vi "All_Data_To_Cluster.vi"(0 "Test":sgl[][](array[numeric]), 1 "Dev":sgl[](array[numeric]), 2 "Inacc":sgl[](array[numeric]), 3 "DIN":string, 4 "HN":string[](array[string]), 5 "HS":sgl[](array[numeric]), 6 "TEMP":string, 7 "TV":sgl[][](array[numeric]), 8 "TSN":string, 9 "HV":sgl[](array[numeric]), 10 "MODE":string, 11 "REP":sgl[](array[numeric]), 13 "AVG":sgl[](array[numeric])) -> (14 "All_data_String":string[][](array[string]), 16 "Test_Data":T1)   [LabVIEW 2019]
uses:
  Test_data.ctl
  Test_load.ctl
  Hardness_test.ctl
  TEST.lvclass
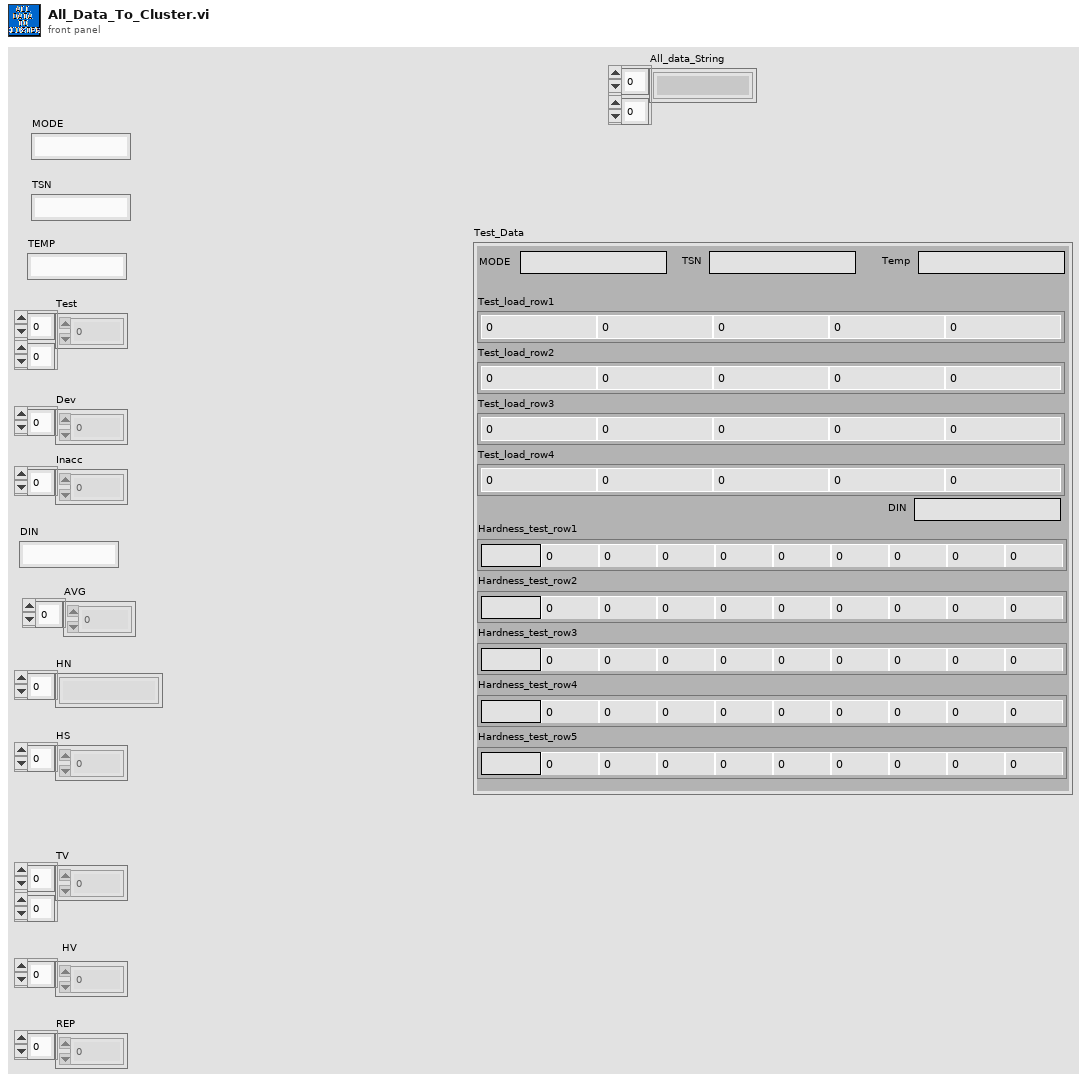
[diagram p1: front panel]
types:
  T1 = typedef "TEST.lvclass/Test_data.ctl" = cluster{"MODE":string, "TSN":string, "Temp":string, "Test_load_row1":T2, "Test_load_row2":T2, "Test_load_row3":T2, "Test_load_row4":T2, "DIN":string, "Hardness_test_row1":T3, "Hardness_test_row2":T3, "Hardness_test_row3":T3, "Hardness_test_row4":T3, "Hardness_test_row5":T3}
  T2 = typedef "TEST.lvclass/Test_load.ctl" = cluster{"TEST1":sgl, "TEST2":sgl, "TEST3":sgl, "DEV":sgl, "INACC":sgl}
  T3 = typedef "TEST.lvclass/Hardness_test.ctl" = cluster{"HN":string, "HS":sgl, "TV1":sgl, "TV2":sgl, "TV3":sgl, "TV4":sgl, "TV5":sgl, "AVG":sgl, "HV":sgl, "REP":sgl}
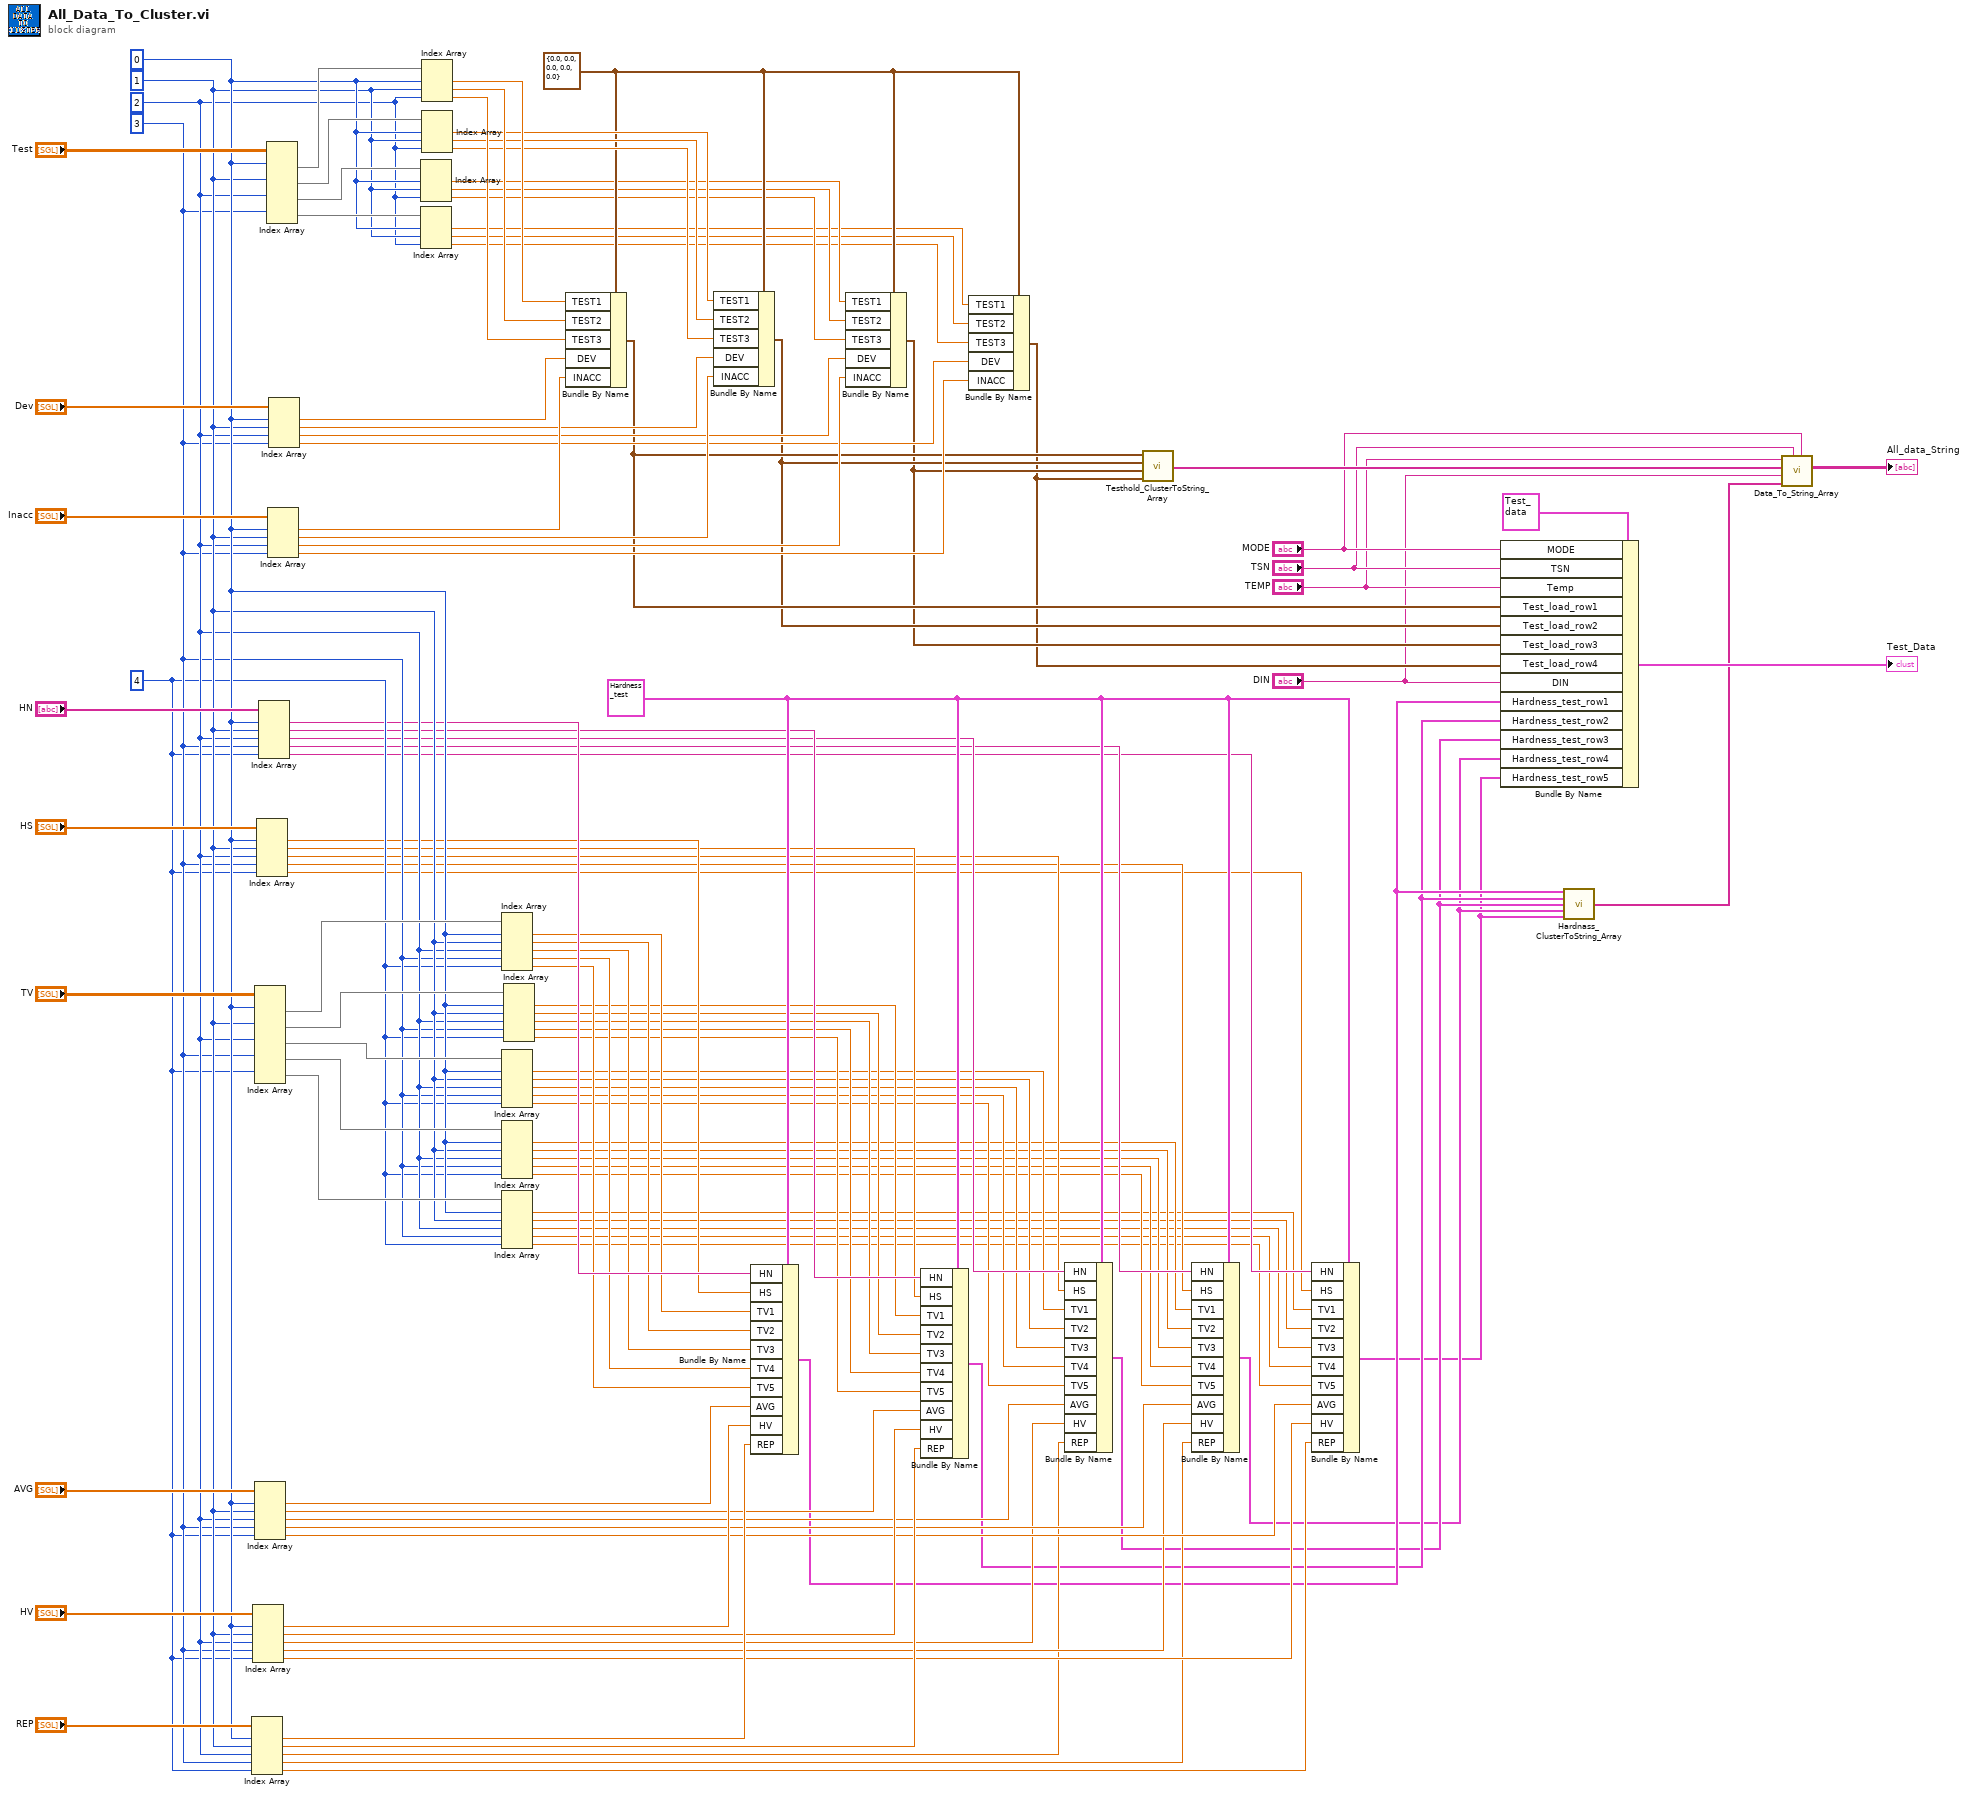
[diagram p0: block diagram]
diagram:
  w64 = T3 {"HN"="", "HS"=0.0, "TV1"=0.0, "TV2"=0.0, "TV3"=0.0, "TV4"=0.0, "TV5"=0.0, "AVG"=0.0, "HV"=0.0, "REP"=0.0} ("Hardness_test")
  w70 = 4
  w98 = T2 {"TEST1"=0.0, "TEST2"=0.0, "TEST3"=0.0, "DEV"=0.0, "INACC"=0.0} ("Test_load")
  w71 = 3 ("索引 (行)")
  w72 = 2 ("索引 (行)")
  w73 = 1 ("索引 (行)")
  w74 = 0 ("索引 (行)")
  n1 = Index Array(array="REP", index #1=w74, index #2=w73, index #3=w72, index #4=w71, index #5=w70) -> (element #1=w65:sgl, element #2=w59:sgl, element #3=w46:sgl, element #4=w45:sgl, element #5=w44:sgl)
  n2 = Index Array(array="HV", index #1=w74, index #2=w73, index #3=w72, index #4=w71, index #5=w70) -> (element #1=w66:sgl, element #2=w60:sgl, element #3=w49:sgl, element #4=w48:sgl, element #5=w47:sgl)
  n3 = Index Array(array="TV", index (row) #1=w74, index (row) #2=w73, index (row) #3=w72, index (row) #4=w71, index (row) #5=w70) -> (element #1=w79:sgl[], element #2=w78:sgl[], element #3=w77:sgl[], element #4=w76:sgl[], element #5=w75:sgl[])  [unwired: 5 in]
  n4 = Index Array(array="AVG", index #1=w74, index #2=w73, index #3=w72, index #4=w71, index #5=w70) -> (element #1=w67:sgl, element #2=w61:sgl, element #3=w52:sgl, element #4=w51:sgl, element #5=w50:sgl)
  n5 = Index Array(array="HS", index #1=w74, index #2=w73, index #3=w72, index #4=w71, index #5=w70) -> (element #1=w68:sgl, element #2=w62:sgl, element #3=w55:sgl, element #4=w54:sgl, element #5=w53:sgl)
  n6 = Index Array(array="HN", index #1=w74, index #2=w73, index #3=w72, index #4=w71, index #5=w70) -> (element #1=w69:string, element #2=w63:string, element #3=w58:string, element #4=w57:string, element #5=w56:string)
  n7 = Index Array(array="Test", index (row) #1=w74, index (row) #2=w73, index (row) #3=w72, index (row) #4=w71) -> (element #1=w110:sgl[], element #2=w109:sgl[], element #3=w108:sgl[], element #4=w107:sgl[])  [unwired: 4 in]
  n8 = Index Array(array="Inacc", index #1=w74, index #2=w73, index #3=w72, index #4=w71) -> (element #1=w102:sgl, element #2=w90:sgl, element #3=w88:sgl, element #4=w86:sgl)
  n9 = Index Array(array="Dev", index #1=w74, index #2=w73, index #3=w72, index #4=w71) -> (element #1=w103:sgl, element #2=w91:sgl, element #3=w89:sgl, element #4=w87:sgl)
  n10 = Index Array(array=w108, index #1=w74, index #2=w73, index #3=w72) -> (element #1=w97:sgl, element #2=w96:sgl, element #3=w95:sgl)
  n11 = Index Array(array=w107, index #1=w74, index #2=w73, index #3=w72) -> (element #1=w94:sgl, element #2=w93:sgl, element #3=w92:sgl)
  n12 = Index Array(array=w110, index #1=w74, index #2=w73, index #3=w72) -> (element #1=w106:sgl, element #2=w105:sgl, element #3=w104:sgl)
  n13 = Index Array(array=w109, index #1=w74, index #2=w73, index #3=w72) -> (element #1=w101:sgl, element #2=w100:sgl, element #3=w99:sgl)
  n14 = Index Array(array=w79, index #1=w74, index #2=w73, index #3=w72, index #4=w71, index #5=w70) -> (element #1=w33:sgl, element #2=w32:sgl, element #3=w31:sgl, element #4=w30:sgl, element #5=w29:sgl)
  n15 = Index Array(array=w77, index #1=w74, index #2=w73, index #3=w72, index #4=w71, index #5=w70) -> (element #1=w23:sgl, element #2=w22:sgl, element #3=w21:sgl, element #4=w20:sgl, element #5=w19:sgl)
  n16 = Index Array(array=w76, index #1=w74, index #2=w73, index #3=w72, index #4=w71, index #5=w70) -> (element #1=w18:sgl, element #2=w17:sgl, element #3=w16:sgl, element #4=w15:sgl, element #5=w14:sgl)
  n17 = Index Array(array=w75, index #1=w74, index #2=w73, index #3=w72, index #4=w71, index #5=w70) -> (element #1=w13:sgl, element #2=w12:sgl, element #3=w11:sgl, element #4=w10:sgl, element #5=w9:sgl)
  n18 = Index Array(array=w78, index #1=w74, index #2=w73, index #3=w72, index #4=w71, index #5=w70) -> (element #1=w28:sgl, element #2=w27:sgl, element #3=w26:sgl, element #4=w25:sgl, element #5=w24:sgl)
  n19 = Bundle By Name(cluster=w98, "TEST1"=w106, "TEST2"=w105, "TEST3"=w104, "DEV"=w103, "INACC"=w102) -> (w42:T2)
  n20 = Bundle By Name(cluster=w98, "TEST1"=w101, "TEST2"=w100, "TEST3"=w99, "DEV"=w91, "INACC"=w90) -> (w41:T2)
  n21 = Bundle By Name(cluster=w64, "HN"=w69, "HS"=w68, "TV1"=w33, "TV2"=w32, "TV3"=w31, "TV4"=w30, "TV5"=w29, "AVG"=w67, "HV"=w66, "REP"=w65) -> (w38:T3)
  n22 = Bundle By Name(cluster=w98, "TEST1"=w97, "TEST2"=w96, "TEST3"=w95, "DEV"=w89, "INACC"=w88) -> (w40:T2)
  n23 = Bundle By Name(cluster=w64, "HN"=w63, "HS"=w62, "TV1"=w28, "TV2"=w27, "TV3"=w26, "TV4"=w25, "TV5"=w24, "AVG"=w61, "HV"=w60, "REP"=w59) -> (w37:T3)
  n24 = Bundle By Name(cluster=w98, "TEST1"=w94, "TEST2"=w93, "TEST3"=w92, "DEV"=w87, "INACC"=w86) -> (w39:T2)
  n25 = Bundle By Name(cluster=w64, "HN"=w58, "HS"=w55, "TV1"=w23, "TV2"=w22, "TV3"=w21, "TV4"=w20, "TV5"=w19, "AVG"=w52, "HV"=w49, "REP"=w46) -> (w36:T3)
  n26 = call "Testhold_ClusterToString_Array.vi"("SLG_Cluster4"=w39, "SLG_Cluster3"=w40, "SLG_Cluster2"=w41, "SLG_Cluster"=w42) -> ("String_Array"=w6:string[])  [unwired: 7 in]
  n27 = Bundle By Name(cluster=w64, "HN"=w57, "HS"=w54, "TV1"=w18, "TV2"=w17, "TV3"=w16, "TV4"=w15, "TV5"=w14, "AVG"=w51, "HV"=w48, "REP"=w45) -> (w35:T3)
  n28 = Bundle By Name(cluster=w64, "HN"=w56, "HS"=w53, "TV1"=w13, "TV2"=w12, "TV3"=w11, "TV4"=w10, "TV5"=w9, "AVG"=w50, "HV"=w47, "REP"=w44) -> (w34:T3)
  n29 = Bundle By Name(cluster=T1 {"MODE"="", "TSN"="", "Temp"="", "Test_load_row1"={"TEST1"=0.0, "TEST2"=0.0, "TEST3"=0.0, "DEV"=0.0, "INACC"=0.0}, "Test_load_row2"={"TEST1"=0.0, "TEST2"=0.0, "TEST3"=0.0, "DEV"=0.0, "INACC"=0.0}, "Test_load_row3"={"TEST1"=0.0, "TEST2"=0.0, "TEST3"=0.0, "DEV"=0.0, "INACC"=0.0}, "Test_load_row4"={"TEST1"=0.0, "TEST2"=0.0, "TEST3"=0.0, "DEV"=0.0, "INACC"=0.0}, "DIN"="", "Hardness_test_row1"={"HN"="", "HS"=0.0, "TV1"=0.0, "TV2"=0.0, "TV3"=0.0, "TV4"=0.0, "TV5"=0.0, "AVG"=0.0, "HV"=0.0, "REP"=0.0}, "Hardness_test_row2"={"HN"="", "HS"=0.0, "TV1"=0.0, "TV2"=0.0, "TV3"=0.0, "TV4"=0.0, "TV5"=0.0, "AVG"=0.0, "HV"=0.0, "REP"=0.0}, "Hardness_test_row3"={"HN"="", "HS"=0.0, "TV1"=0.0, "TV2"=0.0, "TV3"=0.0, "TV4"=0.0, "TV5"=0.0, "AVG"=0.0, "HV"=0.0, "REP"=0.0}, "Hardness_test_row4"={"HN"="", "HS"=0.0, "TV1"=0.0, "TV2"=0.0, "TV3"=0.0, "TV4"=0.0, "TV5"=0.0, "AVG"=0.0, "HV"=0.0, "REP"=0.0}, "Hardness_test_row5"={"HN"="", "HS"=0.0, "TV1"=0.0, "TV2"=0.0, "TV3"=0.0, "TV4"=0.0, "TV5"=0.0, "AVG"=0.0, "HV"=0.0, "REP"=0.0}} ("Cluster8"), "MODE"="MODE", "TSN"="TSN", "Temp"="TEMP", "Test_load_row1"=w42, "Test_load_row2"=w41, "Test_load_row3"=w40, "Test_load_row4"=w39, "DIN"="DIN", "Hardness_test_row1"=w38, "Hardness_test_row2"=w37, "Hardness_test_row3"=w36, "Hardness_test_row4"=w35, "Hardness_test_row5"=w34) -> (→"Test_Data":T1)
  n30 = call "Hardnass_ClusterToString_Array.vi"("Hardness_test"=w38, "Hardness_test 2"=w37, "Hardness_test 3"=w36, "Hardness_test 4"=w35, "Hardness_test 5"=w34) -> ("StringArray"=w7:string[])  [unwired: 10 in]
  n31 = call "Data_To_String_Array.vi"("MODE"="MODE", "TSN"="TSN", "Hardness_string"=w7, "DIN"="DIN", "Test_load_string"=w6, "TEMP"="TEMP") -> ("String_Array"=→"All_data_String":string[][])  [unwired: 5 in]
